vi "Taller 1 punto 2.vi"() -> ()   [LabVIEW 2017]
panel:
  in  "Acción":bool
  in  "Llenado/Vaciado":bool
  in  "Velocidad":bool
  out "Tanque Vacío":bool
  out "Tanque Lleno":bool
  out "Paro":bool
  out "Llenando":bool
  out "Vaciando":bool
  out "Tanque":dbl(slide) scale=0.0..1000.0
  # "TALLER 1, PUNTO 2\nLUZ ANDREA JARAMILLO CASTILLO"
  # "ALTA"
  # "BAJA"
  # "LLENAR"
  # "VACIAR"
  # "CONTINUAR"
  # "PARAR"
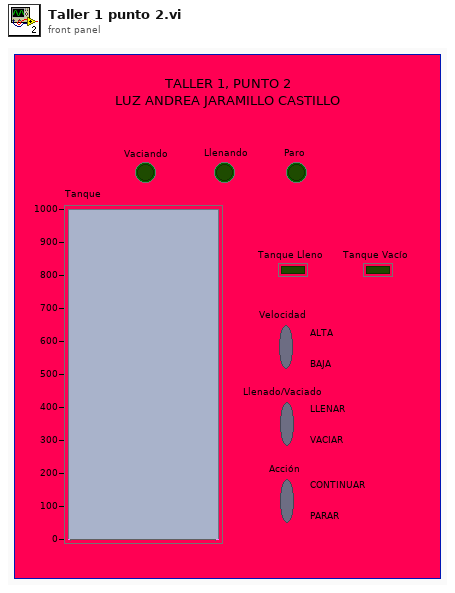
[diagram p1: front panel]
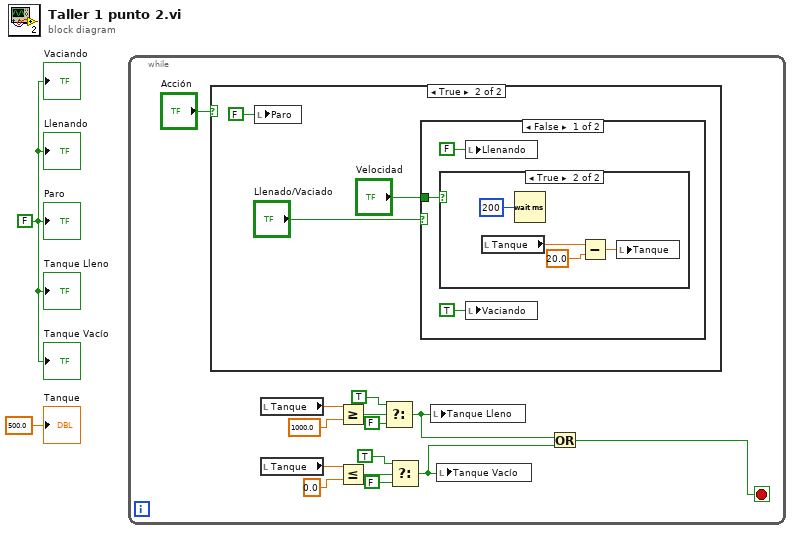
[diagram p0: block diagram]
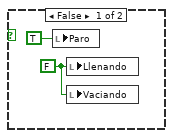
[diagram p2: hidden frame]
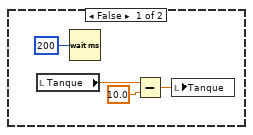
[diagram p3: hidden frame]
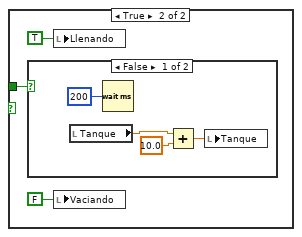
[diagram p4: hidden frame]
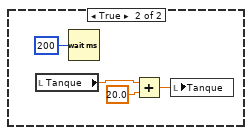
[diagram p5: hidden frame]
diagram:
  w1 = FALSE ("Llenando")
  n1 = while {
    stop <- w3 stop-if-true
    n2 = case shown="True" "Acción" {
      frame False {
        w17 = FALSE ("Llenando")
        n3 = local write "Paro"(TRUE ("Llenando")) -> ()
        n4 = local write "Llenando"(w17) -> ()
        n5 = local write "Vaciando"(w17) -> ()
      }
      frame True {
        n6 = local write "Paro"(FALSE ("Llenando")) -> ()
        n7 = case shown="False" "Llenado/Vaciado" {
          tunnel: "Velocidad" -> [w24 w35]
          frame False {
            n8 = case shown="True" w24 {
              frame False {
                n9 = local read "Tanque"() -> (w28:dbl)
                n10 = Wait (ms)(milliseconds to wait=u32 200) -> ()  [unwired: 1 out]
                n11 = Subtract(x=w28, y=10.0) -> (x-y=w27:dbl)
                n12 = local write "Tanque"(w27) -> ()
              }
              frame True {
                n13 = local read "Tanque"() -> (w32:dbl)
                n14 = Wait (ms)(milliseconds to wait=u32 200) -> ()  [unwired: 1 out]
                n15 = Subtract(x=w32, y=20.0) -> (x-y=w31:dbl)
                n16 = local write "Tanque"(w31) -> ()
              }
            }
            n17 = local write "Llenando"(FALSE ("Llenando")) -> ()
            n18 = local write "Vaciando"(TRUE ("Llenando")) -> ()
          }
          frame True {
            n19 = case shown="False" w35 {
              frame False {
                n20 = local read "Tanque"() -> (w39:dbl)
                n21 = Wait (ms)(milliseconds to wait=u32 200) -> ()  [unwired: 1 out]
                n22 = Add(x=w39, y=10.0) -> (x+y=w38:dbl)
                n23 = local write "Tanque"(w38) -> ()
              }
              frame True {
                n24 = local read "Tanque"() -> (w43:dbl)
                n25 = Wait (ms)(milliseconds to wait=u32 200) -> ()  [unwired: 1 out]
                n26 = Add(x=w43, y=20.0) -> (x+y=w41:dbl)
                n27 = local write "Tanque"(w41) -> ()
              }
            }
            n28 = local write "Llenando"(TRUE ("Llenando")) -> ()
            n29 = local write "Vaciando"(FALSE ("Llenando")) -> ()
          }
        }
      }
    }
    n30 = local read "Tanque"() -> (w15:dbl)
    n31 = local read "Tanque"() -> (w12:dbl)
    n32 = Greater Or Equal?(x=w15, y=1000.0) -> (x >= y?=w11:bool)
    n33 = Less Or Equal?(x=w12, y=0.0) -> (x <= y?=w8:bool)
    n34 = Select(t=TRUE, s=w11, f=FALSE) -> (s? t:f=w5:bool)
    n35 = Select(t=TRUE, s=w8, f=FALSE) -> (s? t:f=w4:bool)
    n36 = local write "Tanque Lleno"(w5) -> ()
    n37 = local write "Tanque Vacío"(w4) -> ()
    n38 = Or(x=w5, y=w4) -> (x .or. y?=w3:bool)
  }
  "Tanque" <- 500.0 ("Tanque")
  "Vaciando" <- w1
  "Paro" <- w1
  "Tanque Lleno" <- w1
  "Tanque Vacío" <- w1
  "Llenando" <- w1
